vi "Straight Movement.vi"(9 "EncoderDevRef":T10={"DevStatus"={"status"=FALSE, "code"=0, "source"=""}, "EncoderIndex"=enum."Invalid", "CounterIndex"=enum."Ctr 1", "DistancePerCount"=2.0, "Decoding Type"=enum."4x"}, 10 "EncoderDevRef 2":T10={"DevStatus"={"status"=FALSE, "code"=0, "source"=""}, "EncoderIndex"=enum."Invalid", "CounterIndex"=enum."Ctr 1", "DistancePerCount"=2.0, "Decoding Type"=enum."4x"}, 11 "RobotDriveDevRef":T2={"DevStatus"={"status"=FALSE, "code"=0, "source"=""}, "Motors[]"=[], "Square Inputs"=FALSE, "Max Output"=1.0, "Isochronous"=FALSE}) -> (3 "Finished?":bool)   [LabVIEW 2012]
uses:
  <vilib>/addons/control/pid/NI_PID_pid.lvlib
  <vilib>/addons/control/pid/pid.llb/PID (DBL).vi
  <vilib>/Rock Robotics/SystemInterfaces/Encoder/FPGA_EncoderIdx.ctl
  <vilib>/Rock Robotics/WPI/Encoder/WPI_EncoderType.ctl
  <vilib>/Rock Robotics/SystemInterfaces/Counter/FPGA_CounterCtrSystemIndex.ctl
  <vilib>/Rock Robotics/WPI/Encoder/WPI_EncoderDevRef.ctl
  <vilib>/Rock Robotics/WPI/PWM/WPI_PWMTransform_ConPane.ctl
  <vilib>/Rock Robotics/SystemInterfaces/Typedef/FPGA_TypedefDigitalModule.ctl
  <vilib>/Rock Robotics/SystemInterfaces/DIO/FPGA_DIOPWMChannel.ctl
  <vilib>/Rock Robotics/WPI/PWM/WPI_PWMDeadband.ctl
  <vilib>/Rock Robotics/WPI/CAN/Jaguar/SubVIs/WPI_CANJaguar_ControlMode.ctl
  <vilib>/Rock Robotics/WPI/MotorControl/WPI_MotorControlDeviceRef.ctl
  <vilib>/Rock Robotics/WPI/RobotDrive/WPI_RobotDriveDevRef.ctl
panel:
  in  "Max Speed":dbl
  in  "Slow-down time":dbl
  in  "Speed-up time":dbl
  in  "Time":dbl
  in  "Spare Correction Time":dbl
  in  "Tolerance":dbl
  in  "Smooth Movment PID gains":T1={"proportional gain (Kc)"=1.0, "integral time (Ti, min)"=0.01, "derivative time (Td, min)"=0.0} {"derivative time (Td, min)" format="%.3f"; "integral time (Ti, min)" format="%.3f"; "proportional gain (Kc)" format="%.3f"}
  in  "Correction PID gains":T1={"proportional gain (Kc)"=1.0, "integral time (Ti, min)"=0.01, "derivative time (Td, min)"=0.0} {"derivative time (Td, min)" format="%.3f"; "integral time (Ti, min)" format="%.3f"; "proportional gain (Kc)" format="%.3f"}
  in  "Distance to Move":dbl
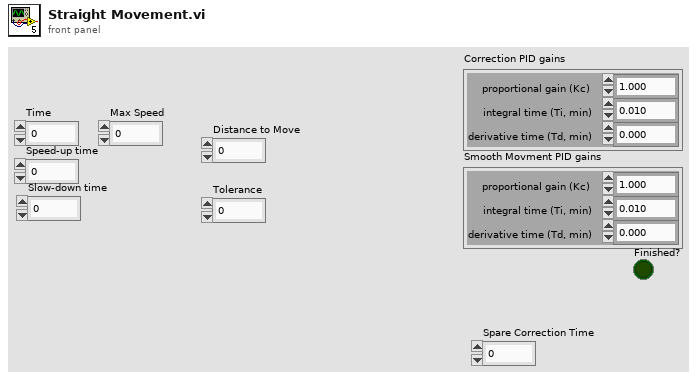
[diagram p1: front panel]
types:
  T1 = cluster{"proportional gain (Kc)":dbl, "integral time (Ti, min)":dbl, "derivative time (Td, min)":dbl}
  T2 = typedef "WPI_RobotDriveDevRef.ctl" = cluster{"DevStatus":errorcluster, "Motors[]":T3[], "Square Inputs":bool, "Max Output":dbl, "Isochronous":bool}
  T3 = typedef "WPI_MotorControlDeviceRef.ctl" = cluster{"DeviceStatus":errorcluster, "Type":enum16{"PWM", "CAN"}, "PWM":cluster{"Digital Module":T4, "PWM Channel":T5, "DeadBand":T6}, "CAN":cluster{"Device Number":u8, "Control Mode":T7, "Semaphore":T8, "Max Vout":dbl}, "Invert":bool, "TransformRef":T9, "InvTransformRef":T9}
  T4 = typedef "FPGA_TypedefDigitalModule.ctl" = enum16{"Digital Module 1", "Digital Module 2"}
  T5 = typedef "FPGA_DIOPWMChannel.ctl" = enum8{"PWM 1", "PWM 2", "PWM 3", "PWM 4", "PWM 5", "PWM 6", "PWM 7", "PWM 8", "PWM 9", "PWM 10", "Invalid"}
  T6 = typedef "WPI_PWMDeadband.ctl" = cluster{"Name":string, "maxPositivePwm":i32, "minPositivePwm":i32, "centerPwm":i32, "maxNegativePwm":i32, "minNegativePwm":i32, "angularRange":u16}
  T7 = typedef "WPI_CANJaguar_ControlMode.ctl" = enum8{"Percent VBus", "Current", "Speed", "Position", "Voltage"}
  T8 = typedef "Semaphore RefNum" = refnum<k1>
  T9 = typedef "WPI_PWMTransform_ConPane.ctl" = refnum<vi>
  T10 = typedef "WPI_EncoderDevRef.ctl" = cluster{"DevStatus":errorcluster, "EncoderIndex":T11, "CounterIndex":T12, "DistancePerCount":dbl, "Decoding Type":T13}
  T11 = typedef "FPGA_EncoderIdx.ctl" = enum8{"Enc 0", "Enc 1", "Enc 2", "Enc 3", "Invalid"}
  T12 = typedef "FPGA_CounterCtrSystemIndex.ctl" = enum8{"Ctr 0", "Ctr 1", "Ctr 2", "Ctr 3", "Ctr 4", "Ctr 5", "Ctr 6", "Ctr 7", "Invalid"}
  T13 = typedef "WPI_EncoderType.ctl" = enum16{"1x", "2x", "4x"}
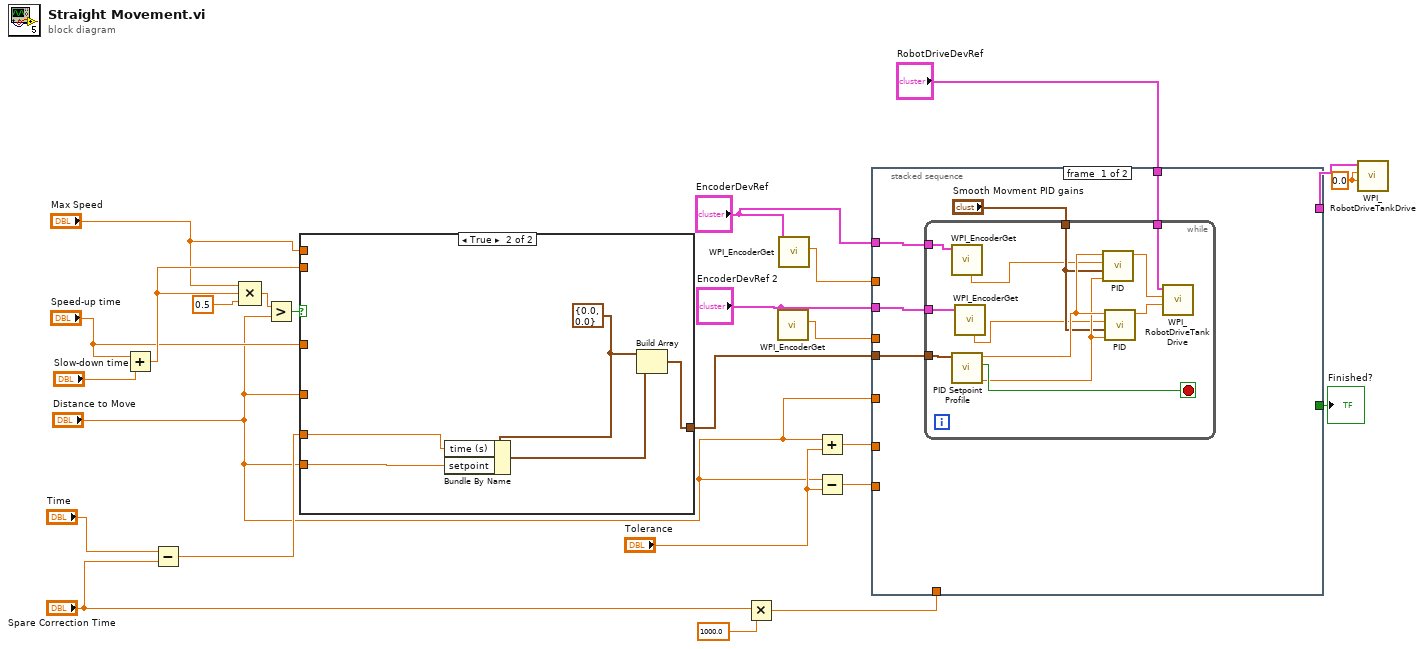
[diagram p0: block diagram]
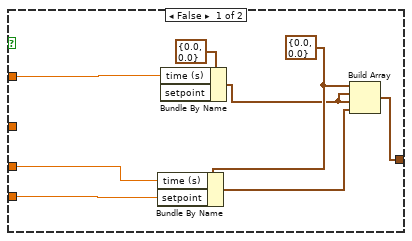
[diagram p2: hidden frame]
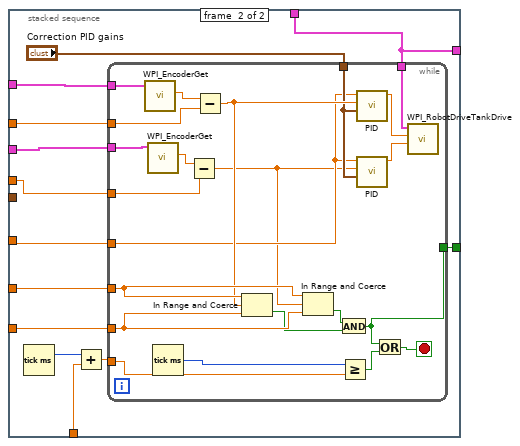
[diagram p3: hidden frame]
diagram:
  w14 = 0.0 ("Left axis value")
  n1 = Add(x="Speed-up time", y="Slow-down time") -> (x+y=w5:dbl)
  n2 = Subtract(x="Time", y="Spare Correction Time") -> (x-y=w6:dbl)
  n3 = Compound Arithmetic op=MULTIPLY("Max Speed", w5, 0.5 ("value")) -> (w4:dbl)
  n4 = Greater?(x=w4, y="Distance to Move") -> (0:w9:bool)
  n5 = case shown="True" w9 {
    tunnel: [w26 w38] -> w8
    tunnel: w6 -> [w29 w34]
    tunnel: "Distance to Move" -> [w30 w36]
    tunnel: w5 -> [_ _]
    tunnel: "Speed-up time" -> [w31 _]
    tunnel: "Max Speed" -> [_ _]
    tunnel: "Distance to Move" -> [_ _]
    frame False {
      w32 = cluster{"time (s)":dbl, "setpoint":dbl} {"time (s)"=0.0, "setpoint"=0.0}
      n6 = Bundle By Name(cluster=w32, "time (s)"=w29, "setpoint"=w30) -> (w28:cluster{"time (s)":dbl, "setpoint":dbl})
      n7 = Bundle By Name(cluster=cluster{"time (s)":dbl, "setpoint":dbl} {"time (s)"=0.0, "setpoint"=0.0}, "time (s)"=w31) -> (w27:cluster{"time (s)":dbl, "setpoint":dbl})  [unwired: 1 in]
      n8 = Build Array(w32, w27, w27, w28) -> (w26:cluster{"time (s)":dbl, "setpoint":dbl}[])
    }
    frame True {
      w37 = cluster{"time (s)":dbl, "setpoint":dbl} {"time (s)"=0.0, "setpoint"=0.0}
      n9 = Bundle By Name(cluster=w37, "time (s)"=w34, "setpoint"=w36) -> (w35:cluster{"time (s)":dbl, "setpoint":dbl})
      n10 = Build Array(w37, w35) -> (w38:cluster{"time (s)":dbl, "setpoint":dbl}[])  [unwired: 1 in]
    }
  }
  n11 = Multiply(x="Spare Correction Time", y=1000.0) -> (x*y=w18:dbl)
  n12 = call <vilib>:"WPI_EncoderGet.vi"("EncoderDevRef"="EncoderDevRef 2") -> ("Distance"=w24:dbl)  [unwired: 5 in, 5 out]
  n13 = call <vilib>:"WPI_EncoderGet.vi"("EncoderDevRef"="EncoderDevRef") -> ("Distance"=w25:dbl)  [unwired: 5 in, 5 out]
  n14 = Add(x="Distance to Move", y="Tolerance") -> (x+y=w17:dbl)
  n15 = Subtract(x="Distance to Move", y="Tolerance") -> (x-y=w16:dbl)
  n16 = stacked-sequence {
    tunnel: w8 -> [w43 _]
    tunnel: "EncoderDevRef 2" -> [w42 w64]
    tunnel: "EncoderDevRef" -> [w41 w65]
    tunnel: w25 -> [_ w63]
    tunnel: w24 -> [_ w62]
    tunnel: "RobotDriveDevRef" -> [w39 w57]
    tunnel: w18 -> [_ w67]
    tunnel: w17 -> [_ w61]
    tunnel: w16 -> [_ w60]
    tunnel: [_ w58] -> w15
    tunnel: [_ w57] -> w13
    tunnel: "Distance to Move" -> [_ w56]
    frame #0 {
      n17 = while {
        tunnel: w43 -> [w52]
        tunnel: w42 -> [w50]
        tunnel: w41 -> [w51]
        tunnel: w39 -> [w47]
        tunnel: "Smooth Movment PID gains" -> [w46]
        stop <- w55 stop-if-true
        n18 = call <vilib>:"WPI_EncoderGet.vi"("EncoderDevRef"=w51) -> ("Rate"=w44:dbl)  [unwired: 5 in, 5 out]
        n19 = call <vilib>:"PID Setpoint Profile.vi"("setpoint profile"=w52) -> ("dt out (s)"=w53:dbl, "profile complete?"=w55:bool, "setpoint"=w54:dbl)  [unwired: 5 in, 1 out]
        n20 = call <vilib>:"WPI_EncoderGet.vi"("EncoderDevRef"=w50) -> ("Rate"=w45:dbl)  [unwired: 5 in, 5 out]
        n21 = call-poly <vilib>:"PID.vi"("dt (s)"=w53, "PID gains"=w46, "process variable"=w44, "setpoint"=w54) -> ("output"=w49:dbl)  [unwired: 6 in, 1 out]
        n22 = call-poly <vilib>:"PID.vi"("dt (s)"=w53, "PID gains"=w46, "process variable"=w45, "setpoint"=w54) -> ("output"=w48:dbl)  [unwired: 6 in, 1 out]
        n23 = call <vilib>:"WPI_RobotDriveTankDrive.vi"("Right axis value"=w48, "Left axis value"=w49, "RobotDriveDevRef"=w47) -> ()  [unwired: 6 in, 3 out]
      }
    }
    frame #1 {
      n24 = Tick Count (ms)() -> (millisecond timer value=w68:u32)
      n25 = Add(x=w68, y=w67) -> (x+y=w66:dbl)
      n26 = while {
        tunnel: w66 -> [w84]
        tunnel: w65 -> [w83]
        tunnel: w64 -> [w82]
        tunnel: w63 -> [w81]
        tunnel: w62 -> [w70]
        tunnel: w61 -> [w79]
        tunnel: w60 -> [w80]
        tunnel: "Correction PID gains" -> [w75]
        tunnel: w57 -> [w74]
        tunnel: [w73] -> w58
        tunnel: w56 -> [w71]
        stop <- w87 stop-if-true
        n27 = call <vilib>:"WPI_EncoderGet.vi"("EncoderDevRef"=w83) -> ("Distance"=w90:dbl)  [unwired: 5 in, 5 out]
        n28 = call <vilib>:"WPI_EncoderGet.vi"("EncoderDevRef"=w82) -> ("Distance"=w72:dbl)  [unwired: 5 in, 5 out]
        n29 = Tick Count (ms)() -> (millisecond timer value=w85:u32)
        n30 = Subtract(x=w72, y=w70) -> (x-y=w69:dbl)
        n31 = Subtract(x=w90, y=w81) -> (x-y=w78:dbl)
        n32 = In Range and Coerce(upper limit=w79, x=w78, lower limit=w80) -> (In Range?=w77:bool)  [unwired: 1 out]
        n33 = In Range and Coerce(upper limit=w79, x=w69, lower limit=w80) -> (In Range?=w76:bool)  [unwired: 1 out]
        n34 = And(x=w76, y=w77) -> (x .and. y?=w73:bool)
        n35 = Greater Or Equal?(x=w85, y=w84) -> (x >= y?=w86:bool)
        n36 = call-poly <vilib>:"PID.vi"("PID gains"=w75, "process variable"=w78, "setpoint"=w71) -> ("output"=w89:dbl)  [unwired: 7 in, 1 out]
        n37 = call-poly <vilib>:"PID.vi"("PID gains"=w75, "process variable"=w69, "setpoint"=w71) -> ("output"=w88:dbl)  [unwired: 7 in, 1 out]
        n38 = Or(x=w73, y=w86) -> (x .or. y?=w87:bool)
        n39 = call <vilib>:"WPI_RobotDriveTankDrive.vi"("Right axis value"=w88, "Left axis value"=w89, "RobotDriveDevRef"=w74) -> ()  [unwired: 6 in, 3 out]
      }
    }
  }
  "Finished?" <- w15
  n40 = call <vilib>:"WPI_RobotDriveTankDrive.vi"("Right axis value"=w14, "Left axis value"=w14, "RobotDriveDevRef"=w13) -> ()  [unwired: 6 in, 3 out]
